vi "Fwd Kenimatics.vi"   [LabVIEW 2013]
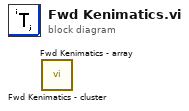
[diagram p0: block diagram]
diagram:
  n1 = call "Fwd Kenimatics - cluster.vi"() -> ()  [unwired: 10 in, 2 out]
  n2 = call "Fwd Kenimatics - array.vi"() -> ()  [unwired: 10 in, 2 out]
